vi "test2-TestFilterJKISMStringQueueVI.vi"(8 "error in (no error)":errorcluster, 11 "TestCase in":refnum<class "testcase-CSMManagementAPI.lvclass">) -> (0 "error out":errorcluster, 3 "TestCase out":refnum<class "testcase-CSMManagementAPI.lvclass">)   [LabVIEW 2017, in "testcase-CSMManagementAPI.lvclass"]
uses:
  testcase-CSMManagementAPI.lvclass
  src/user.lib/_NEVSTOP/Communicable State Machine(CSM)/AdvanceAPI/CSM - Revert Arguments-Safe String.vi
  src/user.lib/_NEVSTOP/Communicable State Machine(CSM)/AdvanceAPI/CSM - Make String Arguments Safe.vi
  src/user.lib/_NEVSTOP/Communicable State Machine(CSM)/AdvanceAPI/CSM - Break Down Multiple States String.vi
  src/user.lib/_NEVSTOP/Communicable State Machine(CSM)/AdvanceAPI/CSM - Compact Multiple States.vi
  src/user.lib/_NEVSTOP/Communicable State Machine(CSM)/AdvanceAPI/CSM - Keywords.vi
  src/user.lib/_NEVSTOP/Communicable State Machine(CSM)/_Polymophic/CSM - Filter Interrupt Broadcasts.vi
  src/user.lib/_NEVSTOP/Communicable State Machine(CSM)/_Polymophic/CSM - Filter Status Broadcasts.vi
  src/user.lib/_NEVSTOP/Communicable State Machine(CSM)/_Polymophic/CSM - Filter Broadcasts.vi
  src/user.lib/_NEVSTOP/Communicable State Machine(CSM)/_Polymophic/CSM - Filter Sync Messages.vi
  src/user.lib/_NEVSTOP/Communicable State Machine(CSM)/_Polymophic/CSM - Filter Async without Reply Messages.vi
  src/user.lib/_NEVSTOP/Communicable State Machine(CSM)/_Polymophic/CSM - Filter Async Messages.vi
  src/user.lib/_NEVSTOP/Communicable State Machine(CSM)/_Polymophic/CSM - Filter Messges.vi
  src/user.lib/_NEVSTOP/Communicable State Machine(CSM)/_Polymophic/CSM - Filter Local States.vi
  src/user.lib/_NEVSTOP/Communicable State Machine(CSM)/_Polymophic/CSM - Filter Duplicated Lines.vi
  src/user.lib/_NEVSTOP/Communicable State Machine(CSM)/AdvanceAPI/CSM - Filter Messages to Non-Existing Modules.vi
  src/user.lib/_NEVSTOP/Communicable State Machine(CSM)/_Shared/Trim Single-line Text.vi
  <vilib>/addons/_JKI Toolkits/VI Tester/TestCase.llb/TestCase.lvclass
  src/user.lib/_NEVSTOP/Communicable State Machine(CSM)/Communicable State Machine.lvlib
  C:/Program Files (x86)/National Instruments/LabVIEW 2017/vi.lib/addons/_JKI Toolkits/VI Tester/TestCase.llb/TestCase.lvclass
panel:
  out "Filter Duplicate Lines No Comments":bool
  out "Filter Duplicate Lines":bool
  out "Filter Duplicate States(Regardless of async/sync/status/interrupt)":bool
  out "Fiter Interrupt Broadcast":bool
  out "Fiter Status Broadcast":bool
  out "Fiter Broadcasts":bool
  out "Filter Messages To Non Existing CSMs":bool
  out "Filter Sync Messages":bool
  out "Filter Async Messages Without Reply":bool
  out "Filter Async Messages":bool
  out "Filter All Messages":bool
  out "Fiter Local States":bool
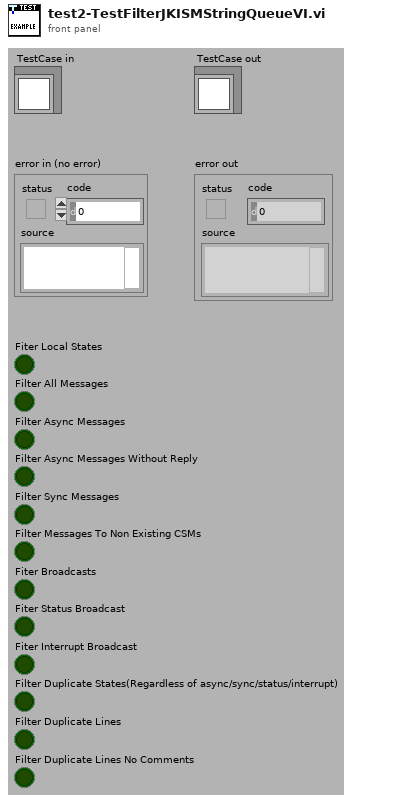
[diagram p1: front panel]
types:
  T1 = enum32{"Invalid", "Standard", "Closed", "Hidden", "Minimized", "Maximized"}
  T2 = enum32{"invalid app kind", "Development System", "Run Time System", "Student Edition", "Embedded LabVIEW", "Evaluation", "Custom"}
  T3 = typedef "Communicable State Machine.lvlib/_CSM_Response Source Message.ctl" = cluster{"‘State":string, "’Arguments":string, "’Error":errorcluster}
  T4 = cluster{"Current VI Reference":refnum<vi>, "Close Panel on Exit?":bool}
  T5 = cluster{"Core":cluster{"Current VI Reference":refnum<vi>, "Close Panel on Exit?":bool}, "Your Boolean data":bool, "Your string data":string}
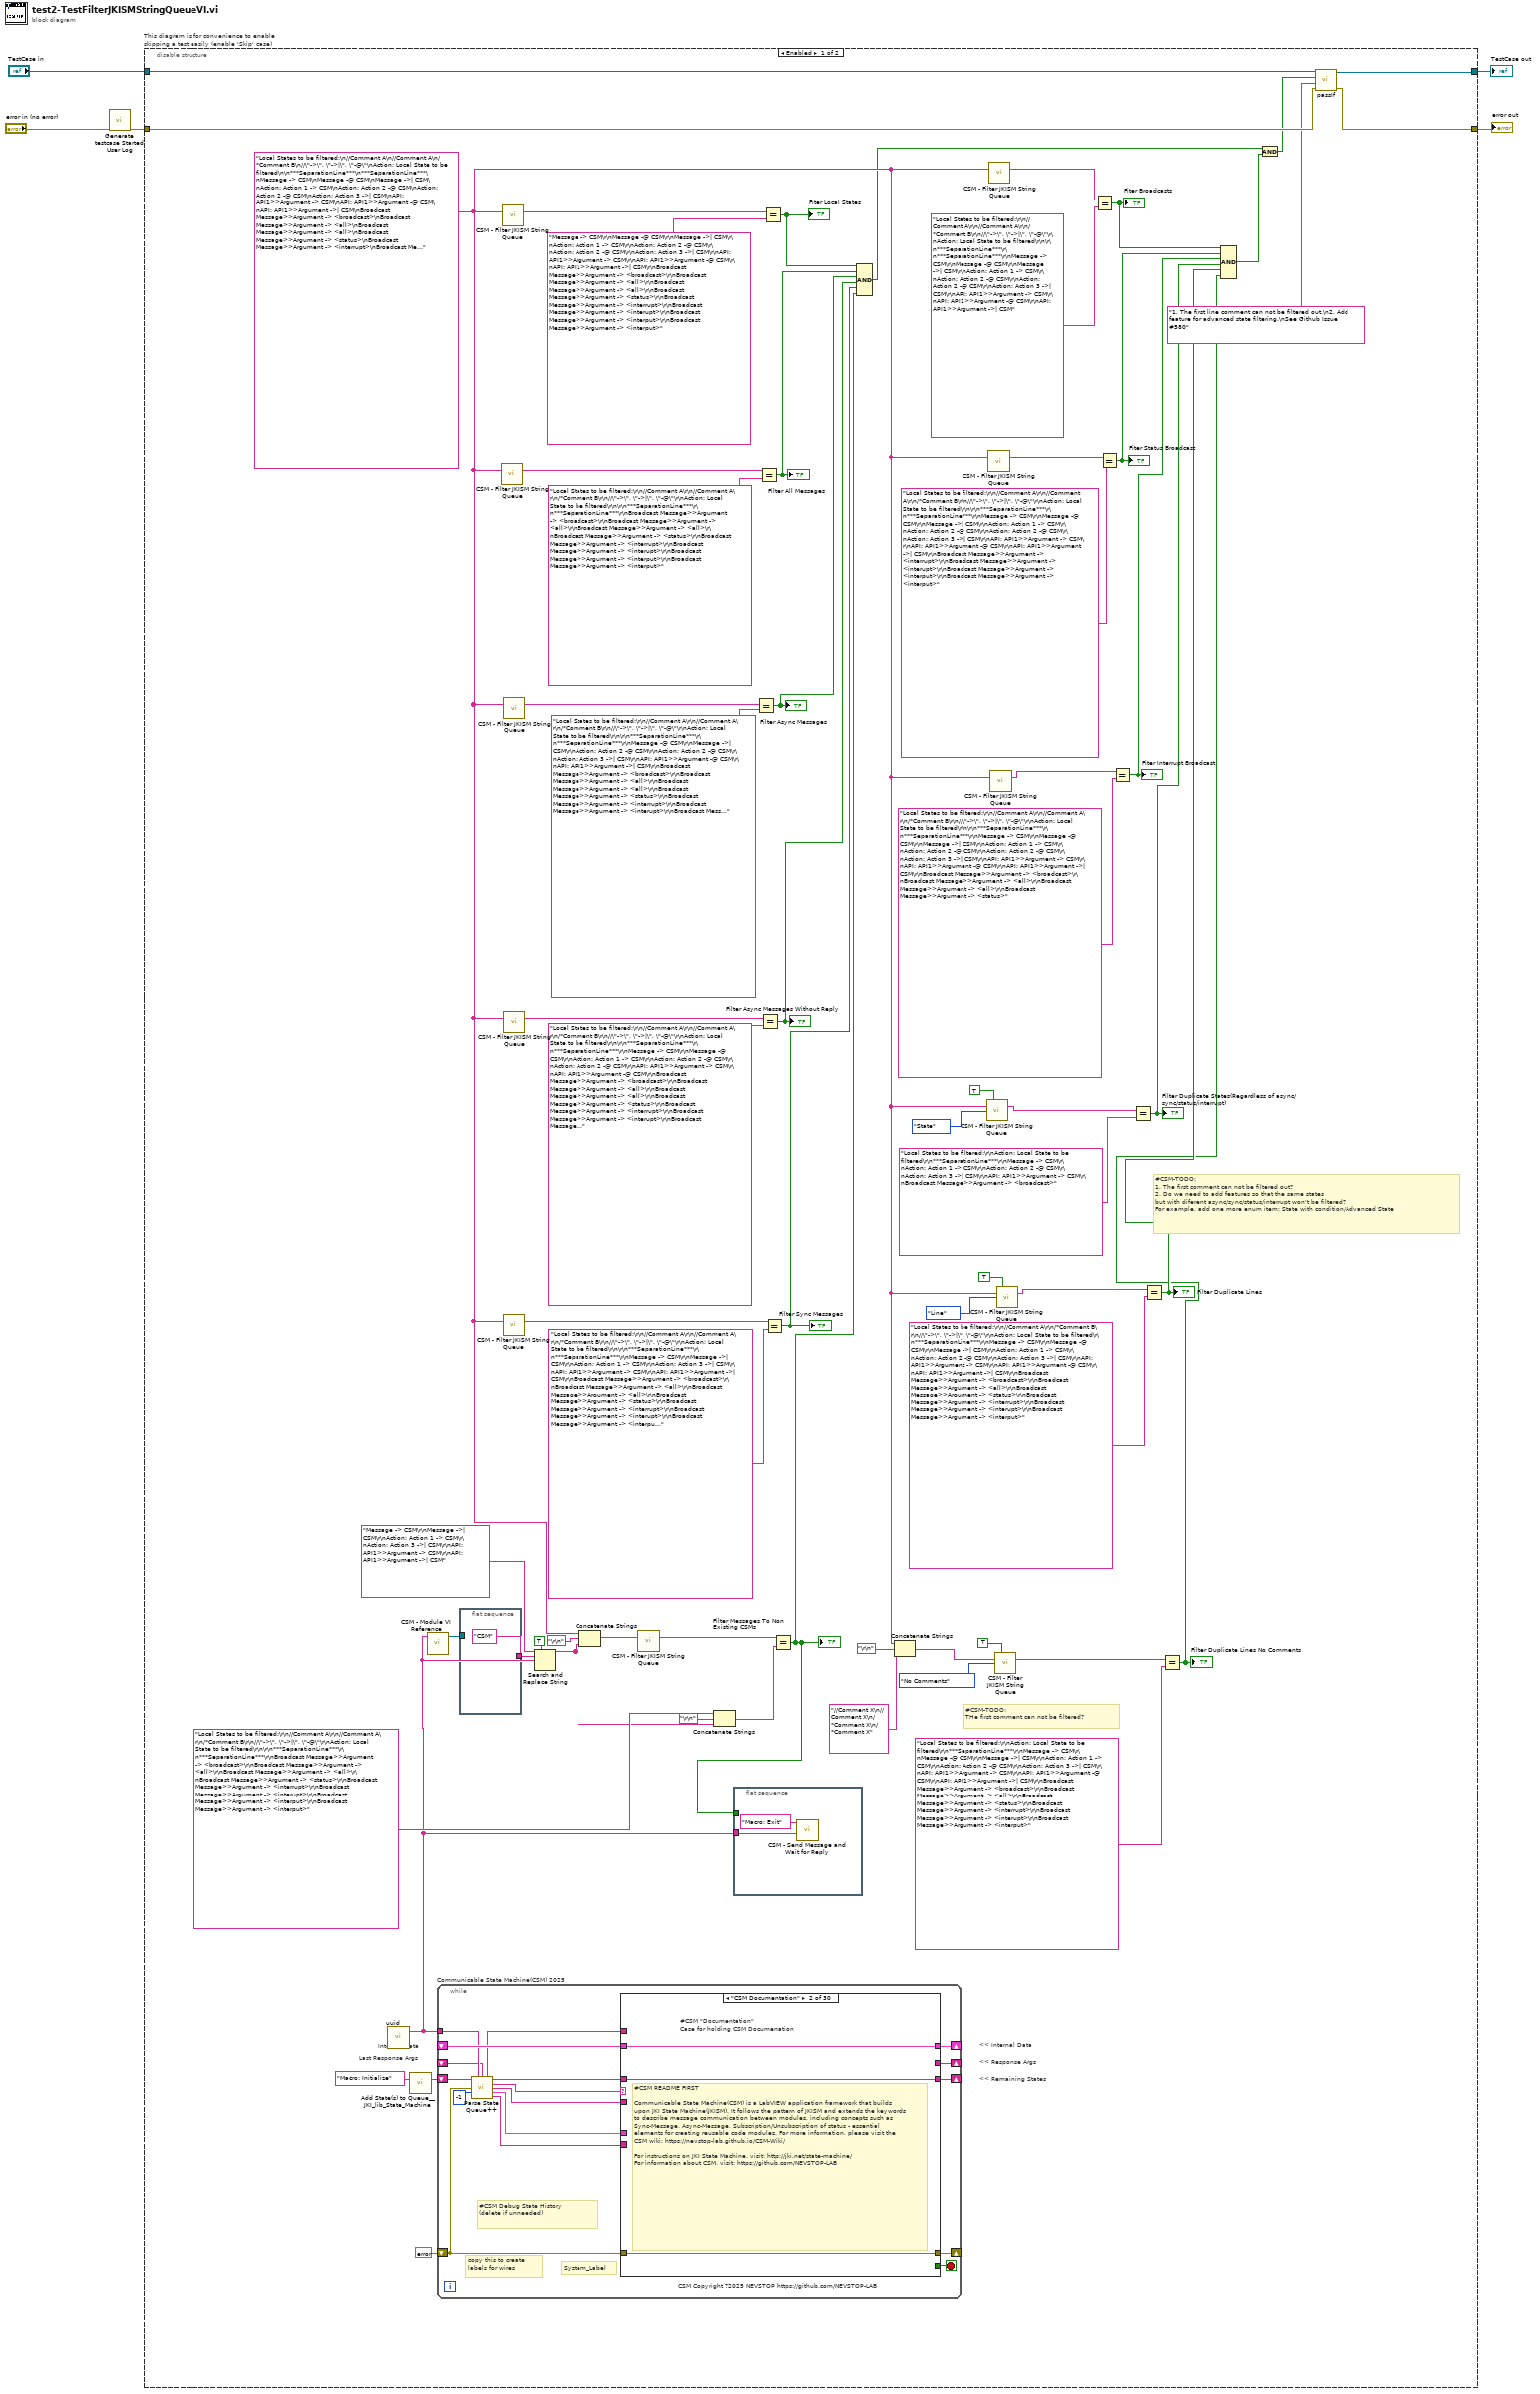
[diagram p0: block diagram]
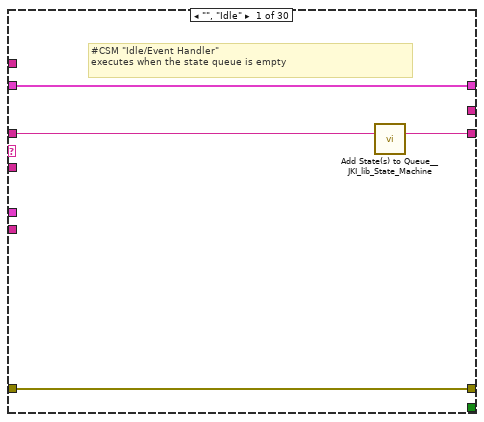
[diagram p2: hidden frame]
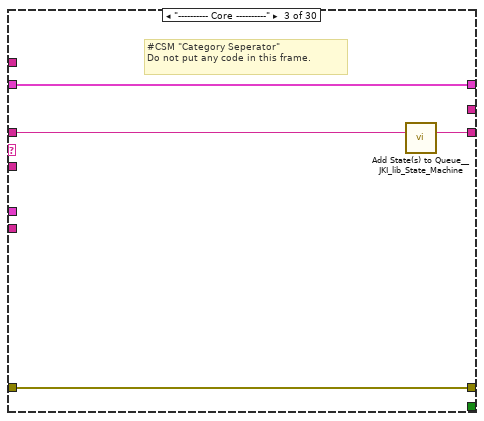
[diagram p3: hidden frame]
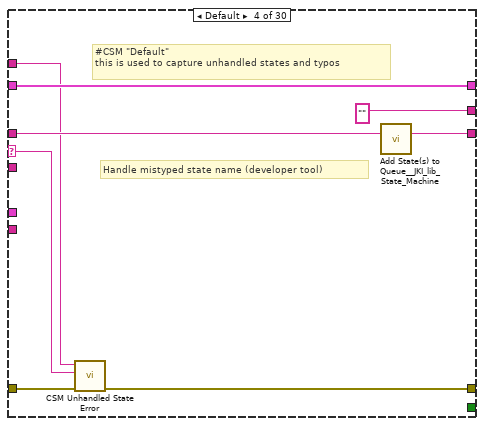
[diagram p4: hidden frame]
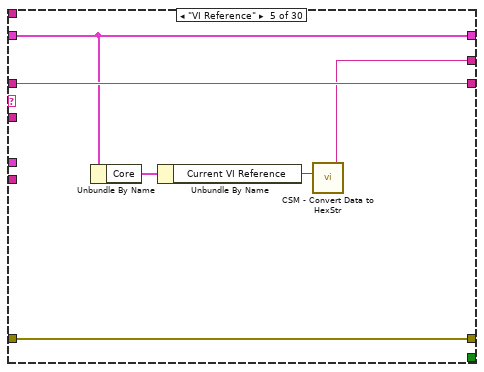
[diagram p5: hidden frame]
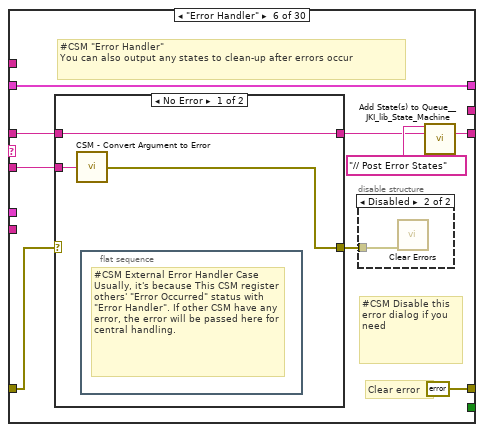
[diagram p6: hidden frame]
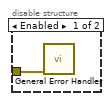
[diagram p7: hidden frame]
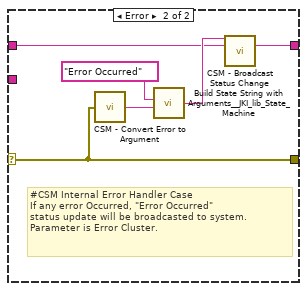
[diagram p8: hidden frame]
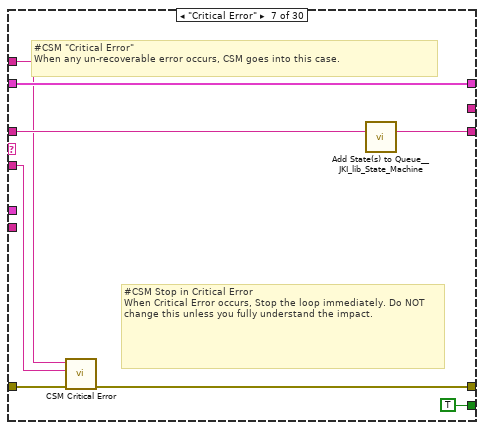
[diagram p9: hidden frame]
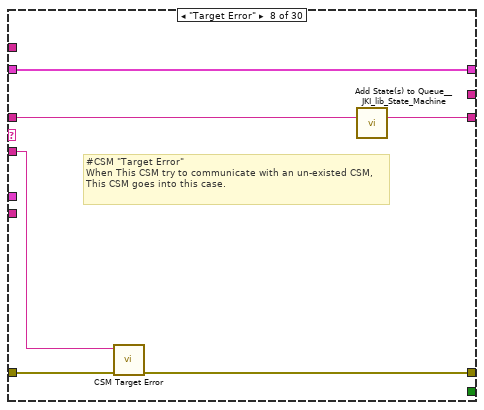
[diagram p10: hidden frame]
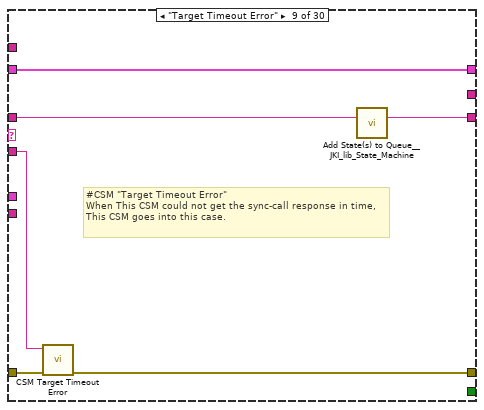
[diagram p11: hidden frame]
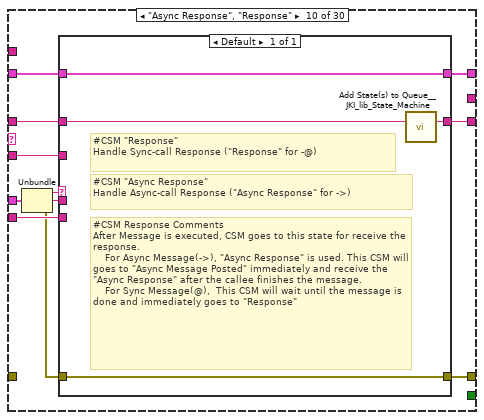
[diagram p12: hidden frame]
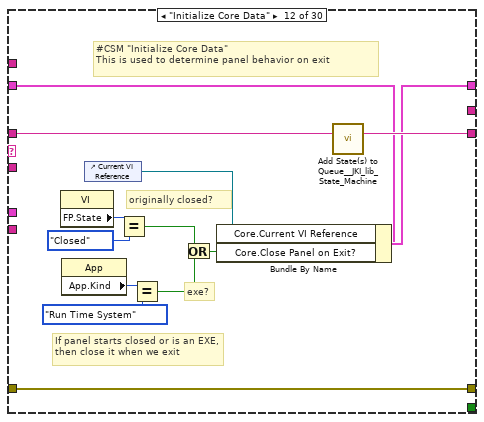
[diagram p14: hidden frame]
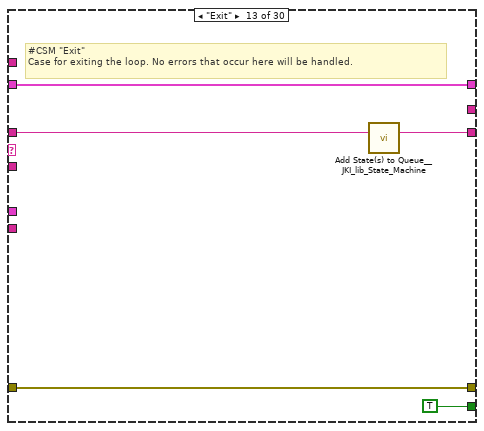
[diagram p15: hidden frame]
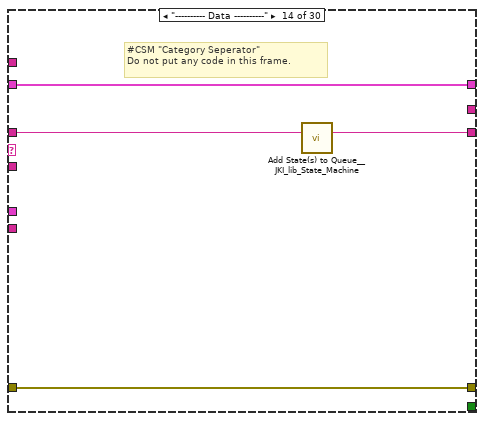
[diagram p16: hidden frame]
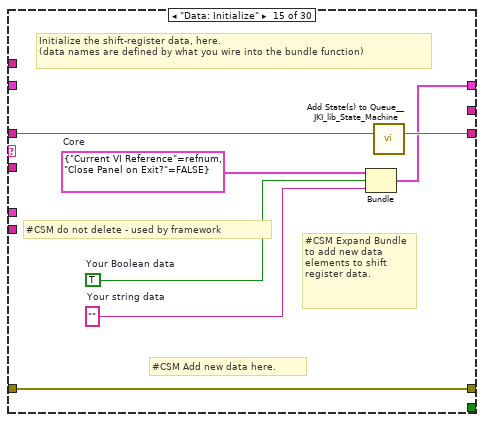
[diagram p17: hidden frame]
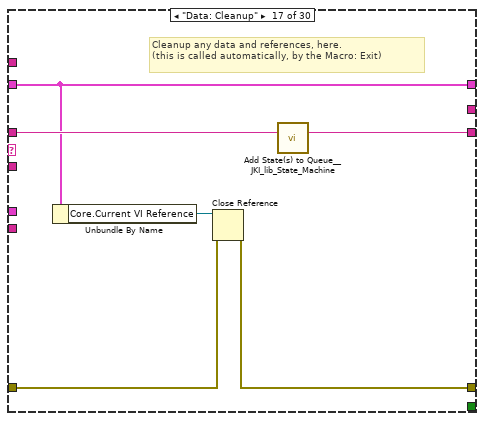
[diagram p19: hidden frame]
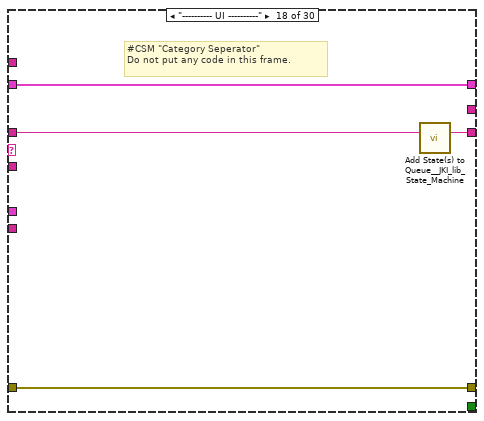
[diagram p20: hidden frame]
diagram:
  n1 = call "Generate testcase Started User Log.vi"("Error In"="error in (no error)") -> ("error out"=w1:errorcluster)  [unwired: 10 in]
  n2 = disable-structure "This diagram is for convenience to enable skipping a test easily (enable 'Skip' case)" shown="Enabled" {
    disable-tunnel: "TestCase in" -> [w32 w353]
    disable-tunnel: [w33 w351] -> w2
    disable-tunnel: [w30 w352] -> w4
    disable-tunnel: w1 -> [w31 w350]
    frame Enabled {
      w38 = "Local States to be filtered:\n//Comment A\n//Comment A\n/*Comment B\n//\"->\", \"->|\", \"-@\"\nAction: Local State to be filtered\n\n***SeparationLine***\n***SeparationLine***\nMessage -> CSM\nMessage -@ CSM\nMessage ->| CSM\nAction: Action 1 -> CSM\nAction: Action 2 -@ CSM\nAction: Action 2 -@ CSM\nAction: Action 3 ->| CSM\nAPI: API1>>Argument -> CSM\nAPI: API1>>Argument -@ CSM\nAPI: API1>>Argument ->| CSM\nBroadcast Message>>Argument -> <broadcast>\nBroadcast Message>>Argument -> <all>\nBroadcast Message>>Argument -> <all>\nBroadcast Message>>Argument -> <status>\nBroadcast Message>>Argument -> <interrupt>\nBroadcast Message>>Argument -> <interupt>\nBroadcast Message>>Argument -> <interput>\nBroadcast Message>>Argument -> <interput>" ("States In")
      # "Last Response Args"
      # "Internal Data"
      # "<< Internal Data"
      # "<< Response Args"
      # "<< Remaining States"
      # "#CSM-TODO:\nTHe first comment can not be filtered?"
      # "#CSM-TODO:\n1. The first comment can not be filtered out?\n2. Do we need to add features so that the same states \nbut with diferent async/sync/status/interrupt won't be filtered?\nFor example, add one more enum item: State with condition/Advanced State"
      n3 = call "uuid.vi"() -> ("UUID"=w7:string)  [unwired: 11 in]
      n4 = call <vilib>:"Add State(s) to Queue__JKI_lib_State_Machine.vi"("State(s) in (\"\")"="Macro: Initialize" ("Init State(\"Macro: Initialize\")")) -> ("States Out"=w11:string)  [unwired: 14 in]
      n5 = call "CSM - Module VI Reference.vi"("CSM Name"=w7) -> ("CSM Module VIRef"=w8:refnum<vi>)  [unwired: 9 in, 1 out]
      n6 = while "Communicable State Machine(CSM) 2025" {
        shift-right: [w87] -> _
        shift-left: _ -> [w86]
        shift-right: [w90] -> _
        shift-left: errorcluster {"status"=FALSE, "code"=0, "source"=""} ("error out") -> [w85]
        shift-right: [w89] -> _
        shift-left: w11 -> [w91]
        tunnel: w7 -> [w83]
        shift-right: [w84] -> _
        shift-left: _ -> [w77]
        stop <- w88 stop-if-true
        # "#CSM Debug State History\n(delete if unneeded)"
        # "copy this to create labels for wires"
        # "System_Label"
        # "CSM Copyright ?2025 NEVSTOP https://github.com/NEVSTOP-LAB"
        n7 = call "Parse State Queue++.vi"("State Queue"=w91, "Name (\"\" to Use UUID)"=w83, "Response Arguments"=w77, "Previous Error"=w85, "Dequeue (1 ms)"=-1 ("Timeout")) -> ("Name Used"=w78:string, "Remaining States"=w92:string, "Current State"=w82:string, "Arguments"=w81:string, "Additional Information"=w80:T3, "Source CSM"=w79:string)  [unwired: 5 in]
        n8 = case shown="\"CSM Documentation\"" w82 {
          selector: w82 -> [_ _ _ w106 _ _ _ _ _ _ _ _ _ _ _ _ _ _ _ _ _ _ _ _ _ _ _ _ _ _]
          tunnel: w92 -> [w93 w98 w103 w110 w116 w122 w143 w149 w155 w163 w174 w188 w193 w197 w204 w206 w213 w217 w221 w227 w242 w311 w316 w323 w325 w329 w334 w341 w345 w349]
          tunnel: w81 -> [_ _ _ _ _ w121 w139 w148 w153 w162 _ _ _ _ _ _ _ _ _ w222 w236 _ _ _ _ _ w332 _ _ _]
          tunnel: w86 -> [w94 w97 w100 w108 w115 w125 w144 w150 w156 w165 w173 w181 w191 w194 _ w205 w208 w214 w219 w225 w238 w308 w313 w320 w324 w328 w333 w338 w342 w346]
          tunnel: [w95 w99 w101 w104 w117 errorcluster {"status"=FALSE, "code"=0, "source"=""} ("error out") w140 w146 w152 w168 w175 w185 w190 w195 w201 w207 w209 w215 w218 w223 w239 w309 w314 w321 w326 w330 w335 w339 w343 w347] -> w90
          tunnel: w85 -> [w95 w99 w101 w111 w117 w123 w145 w147 w154 _ w175 w185 w190 w195 w201 w207 w210 w215 w218 w224 w240 w309 w314 w321 w326 w330 w335 w339 w343 w347]
          tunnel: [w96 w98 w102 w109 w116 w118 w142 w151 w157 w164 w174 w187 w192 w196 w203 w206 w212 w216 w220 w226 w241 w310 w315 w322 w325 w329 w334 w340 w344 w348] -> w89
          tunnel: [_ _ _ _ _ _ TRUE _ _ _ _ _ TRUE _ _ _ _ _ _ _ _ _ _ _ _ _ _ _ _ _] -> w88
          tunnel: [w94 w97 w100 w108 w115 w125 w144 w150 w156 w166 w173 w186 w191 w194 w202 w205 w208 w214 w219 w225 w238 w308 w313 w320 w324 w328 w333 w338 w342 w346] -> w87
          tunnel: w79 -> [_ _ _ _ _ _ _ _ _ w160 _ _ _ _ _ _ _ _ _ _ _ _ _ _ _ _ _ _ _ _]
          tunnel: w80 -> [_ _ _ _ _ _ _ _ _ w167 _ _ _ _ _ _ _ _ _ _ _ _ _ _ _ _ _ _ _ _]
          tunnel: [_ _ _ "" w112 _ _ _ _ _ _ _ _ _ _ _ _ _ _ _ _ _ _ _ _ "API1 Response" w331 _ _ _] -> w84
          tunnel: w78 -> [_ _ _ w105 _ _ w138 _ _ _ _ _ _ _ _ _ _ _ _ _ _ _ _ _ _ _ _ _ _ _]
          frame "", "Idle" {
            # "#CSM \"Idle/Event Handler\"\nexecutes when the state queue is empty"
            n9 = call <vilib>:"Add State(s) to Queue__JKI_lib_State_Machine.vi"("State(s) in (\"\")"=w93) -> ("States Out"=w96:string)  [unwired: 14 in]
          }
          frame "CSM Documentation" {
            # "#CSM README FIRST\n\nCommunicable State Machine(CSM) is a LabVIEW application framework that builds upon JKI State Machine(JKISM). It follows the pattern of JKISM and extends the keywords to describe message communication between modules, including concepts such as Sync-Message, Async-Message, Subscription/Unsubscription of status - essential elements for creating reusable code modules. For more information, please visit the CSM wiki: https://nevstop-lab.github.io/CSM-Wiki/\n\nFor instructions on JKI State Machine, visit: http://jki.net/state-machine/\nFor information about CSM, visit: https://github.com/NEVSTOP-LAB"
            # "#CSM \"Documentation\"\nCase for holding CSM Documenation"
          }
          frame "---------- Core ----------" {
            # "#CSM \"Category Seperator\"\nDo not put any code in this frame."
            n10 = call <vilib>:"Add State(s) to Queue__JKI_lib_State_Machine.vi"("State(s) in (\"\")"=w103) -> ("States Out"=w102:string)  [unwired: 14 in]
          }
          frame Default {
            # "#CSM \"Default\"\nthis is used to capture unhandled states and typos"
            # "Handle mistyped state name (developer tool)"
            n11 = call "CSM Unhandled State Error.vi"("error in (no error)"=w111, "Undefined State"=w106, "CSM Name"=w105) -> ("error out"=w104:errorcluster)  [unwired: 8 in]
            n12 = call <vilib>:"Add State(s) to Queue__JKI_lib_State_Machine.vi"("State(s) in (\"\")"=w110) -> ("States Out"=w109:string)  [unwired: 14 in]
          }
          frame "VI Reference" {
            n13 = Unbundle By Name(w115) -> ("Core"=w114:T4)
            n14 = Unbundle By Name(w114) -> ("Current VI Reference"=w113:refnum<vi>)
            n15 = call "CSM - Convert Data to HexStr.vi"("Variant"=w113) -> ("HEX String (0-9,A-F)"=w112:string)  [unwired: 8 in]
          }
          frame "Error Handler" {
            # "#CSM Disable this error dialog if you need"
            # "#CSM \"Error Handler\"\nYou can also output any states to clean-up after errors occur"
            # "Clear error"
            n16 = case shown="No Error" w123 {
              selector: w123 -> [_ w132]
              tunnel: [w131 w134] -> w119
              tunnel: w122 -> [w131 w133]
              tunnel: w121 -> [w130 _]
              tunnel: [w129 w132] -> w124
              frame No Error {
                n17 = call "CSM - Convert Argument to Error.vi"("Argument"=w130) -> ("Error"=w129:errorcluster)  [unwired: 4 in]
                n18 = flat-sequence {
                  frame #0 {
                    # "#CSM External Error Handler Case\nUsually, it's because This CSM register others' \"Error Occurred\" status with \"Error Handler\". If other CSM have any error, the error will be passed here for central handling."
                  }
                }
              }
              frame Error {
                # "#CSM Internal Error Handler Case \nIf any error Occurred, \"Error Occurred\" \nstatus update will be broadcasted to system.\nParameter is Error Cluster."
                n19 = call "CSM - Convert Error to Argument.vi"("Error"=w132) -> ("Argument"=w136:string)  [unwired: 4 in]
                n20 = call <vilib>:"Build State String with Arguments__JKI_lib_State_Machine.vi"("Arguments (\"\")"=w136, "State"="Error Occurred" ("Status with Arguments")) -> ("State with Arguments"=w135:string)  [unwired: 4 in]
                n21 = call "CSM - Broadcast Status Change.vi"("Status With Arguments"=w135, "State Queue"=w133) -> ("Remaining States"=w134:string)  [unwired: 13 in]
              }
            }
            n22 = disable-structure shown="Disabled" {
              disable-tunnel: w124 -> [w127 w128]
              frame Enabled {
                n23 = call <vilib>:"General Error Handler.vi"("error in (no error)"=w127) -> ()  [unwired: 10 in, 5 out]
              }
              frame Disabled {
                n24 = call <vilib>:"Clear Errors.vi"("error in (no error)"=w128) -> ()  [unwired: 5 in, 2 out]
              }
            }
            n25 = call <vilib>:"Add State(s) to Queue__JKI_lib_State_Machine.vi"("State(s) in Front (\"\")"="// Post Error States", "State(s) in (\"\")"=w119) -> ("States Out"=w118:string)  [unwired: 13 in]
          }
          frame "Critical Error" {
            # "#CSM Stop in Critical Error\nWhen Critical Error occurs, Stop the loop immediately. Do NOT change this unless you fully understand the impact."
            # "#CSM \"Critical Error\"\nWhen any un-recoverable error occurs, CSM goes into this case."
            n26 = call "CSM Critical Error.vi"("error in (no error)"=w145, "Arugments (As Reason)"=w139, "CSM Name"=w138) -> ("error out"=w140:errorcluster)  [unwired: 8 in]
            n27 = call <vilib>:"Add State(s) to Queue__JKI_lib_State_Machine.vi"("State(s) in (\"\")"=w143) -> ("States Out"=w142:string)  [unwired: 14 in]
          }
          frame "Target Error" {
            # "#CSM \"Target Error\"\nWhen This CSM try to communicate with an un-existed CSM, This CSM goes into this case."
            n28 = call "CSM Target Error.vi"("error in (no error)"=w147, "Arguments (As CSM Name)"=w148) -> ("error out"=w146:errorcluster)  [unwired: 9 in]
            n29 = call <vilib>:"Add State(s) to Queue__JKI_lib_State_Machine.vi"("State(s) in (\"\")"=w149) -> ("States Out"=w151:string)  [unwired: 14 in]
          }
          frame "Target Timeout Error" {
            # "#CSM \"Target Timeout Error\"\nWhen This CSM could not get the sync-call response in time, This CSM goes into this case."
            n30 = call "CSM Target Timeout Error.vi"("error in (no error)"=w154, "Arguments (As CSM Name)"=w153) -> ("error out"=w152:errorcluster)  [unwired: 9 in]
            n31 = call <vilib>:"Add State(s) to Queue__JKI_lib_State_Machine.vi"("State(s) in (\"\")"=w155) -> ("States Out"=w157:string)  [unwired: 14 in]
          }
          frame "Async Response", "Response" {
            n32 = Unbundle(w167) -> ("‘State"=w161:string, "’Arguments"=w159:string, "’Error"=w158:errorcluster)
            n33 = case shown="Default" w161 {
              tunnel: [w172] -> w168
              tunnel: w158 -> [w172]
              tunnel: [w171] -> w166
              tunnel: w165 -> [w171]
              tunnel: [w169] -> w164
              tunnel: w163 -> [w170]
              tunnel: w162 -> [_]
              tunnel: w160 -> [_]
              tunnel: w159 -> [_]
              frame Default {
                # "#CSM Response Comments\nAfter Message is executed, CSM goes to this state for receive the response.\n    For Async Message(->), \"Async Response\" is used. This CSM will goes to \"Async Message Posted\" immediately and receive the \"Async Response\" after the callee finishes the message.\n    For Sync Message(@),  This CSM will wait until the message is done and immediately goes to \"Response\""
                # "#CSM \"Async Response\"\nHandle Async-call Response (\"Async Response\" for ->)"
                # "#CSM \"Response\"\nHandle Sync-call Response (\"Response\" for -@)"
                n34 = call <vilib>:"Add State(s) to Queue__JKI_lib_State_Machine.vi"("State(s) in (\"\")"=w170) -> ("States Out"=w169:string)  [unwired: 14 in]
              }
            }
          }
          frame "Async Message Posted" {
            # "#CSM \"Async Message Posted\"\nAfter Async Message is posted (-> or ->| ), CSM goes to this state for post-action.\nYou can use Argument - State to tell which Async Message is called."
          }
          frame "Initialize Core Data" {
            # "#CSM \"Initialize Core Data\"\nThis is used to determine panel behavior on exit"
            # "originally closed?"
            # "exe?"
            # "If panel starts closed or is an EXE, then close it when we exit"
            n35 = property class="VI"() -> ("FP.State"=w178:T1)  [unwired: 2 in, 2 out]
            n36 = property class="App"() -> ("App.Kind"=w184:T2)  [unwired: 2 in, 2 out]
            n37 = control-ref of="Current VI Reference"() -> (w179:refnum<vi>)
            n38 = Equal?(x=w178, y=T1."Closed" ("Front Panel Window:State")) -> (x = y?=w176:bool)
            n39 = Equal?(x=w184, y=T2."Run Time System" ("Application:Kind")) -> (x = y?=w182:bool)
            n40 = Or(x=w176, y=w182) -> (x .or. y?=w180:bool)
            n41 = Bundle By Name(cluster=w181, "Core.Current VI Reference"=w179, "Core.Close Panel on Exit?"=w180) -> (w186:T5)
            n42 = call <vilib>:"Add State(s) to Queue__JKI_lib_State_Machine.vi"("State(s) in (\"\")"=w188) -> ("States Out"=w187:string)  [unwired: 14 in]
          }
          frame "Exit" {
            # "#CSM \"Exit\"\nCase for exiting the loop. No errors that occur here will be handled."
            n43 = call <vilib>:"Add State(s) to Queue__JKI_lib_State_Machine.vi"("State(s) in (\"\")"=w193) -> ("States Out"=w192:string)  [unwired: 14 in]
          }
          frame "---------- Data ----------" {
            # "#CSM \"Category Seperator\"\nDo not put any code in this frame."
            n44 = call <vilib>:"Add State(s) to Queue__JKI_lib_State_Machine.vi"("State(s) in (\"\")"=w197) -> ("States Out"=w196:string)  [unwired: 14 in]
          }
          frame "Data: Initialize" {
            w198 = T4 {"Current VI Reference"=refnum, "Close Panel on Exit?"=FALSE}  # Core
            w200 = TRUE  # Your Boolean data
            w199 = ""  # Your string data
            # "#CSM do not delete - used by framework"
            # "#CSM Expand Bundle to add new data elements to shift register data."
            # "#CSM Add new data here."
            # "Initialize the shift-register data, here.\n(data names are defined by what you wire into the bundle function)"
            n45 = Bundle("Core"=w198, "Your Boolean data"=w200, "Your string data"=w199) -> (w202:T5)  [unwired: 1 in]
            n46 = call <vilib>:"Add State(s) to Queue__JKI_lib_State_Machine.vi"("State(s) in (\"\")"=w204) -> ("States Out"=w203:string)  [unwired: 14 in]
          }
          frame "Data: Update Indicators" {
          }
          frame "Data: Cleanup" {
            # "Cleanup any data and references, here.\n(this is called automatically, by the Macro: Exit)"
            n47 = Unbundle By Name(w208) -> ("Core.Current VI Reference"=w211:refnum<vi>)
            n48 = Close Reference(reference=w211, error in (no error)=w210) -> (error out=w209:errorcluster)
            n49 = call <vilib>:"Add State(s) to Queue__JKI_lib_State_Machine.vi"("State(s) in (\"\")"=w213) -> ("States Out"=w212:string)  [unwired: 14 in]
          }
          frame "---------- UI ----------" {
            # "#CSM \"Category Seperator\"\nDo not put any code in this frame."
            n50 = call <vilib>:"Add State(s) to Queue__JKI_lib_State_Machine.vi"("State(s) in (\"\")"=w217) -> ("States Out"=w216:string)  [unwired: 14 in]
          }
          frame "UI: Initialize" {
            # "#CSM \"UI: Initialize\"\nInitialize the User Interface, here.\n(this is called automatically, by the Macro: Init)"
            n51 = call <vilib>:"Add State(s) to Queue__JKI_lib_State_Machine.vi"("State(s) in (\"\")"=w221) -> ("States Out"=w220:string)  [unwired: 14 in]
          }
          frame "UI: Cursor Set" {
            # "#CSM \"UI: Cursor Set\"\nSet and Unset Cursor Busy.\n(Usage: \"UI: Cursor Set >> Busy|Idle\")"
            # "Argument"
            n52 = disable-structure shown="TARGET_TYPE!=Windows" {
              disable-tunnel: w224 -> [w230 w235]
              disable-tunnel: [w229 w235] -> w223
              disable-tunnel: w222 -> [w228 _]
              frame condition #0 (active) {
                n53 = case shown="\"Idle\", Default" w228 {
                  tunnel: w230 -> [w232 w234]
                  tunnel: [w231 w233] -> w229
                  frame "Idle", Default {
                    n54 = call <vilib>:"Unset Busy.vi"("error in (no error)"=w232) -> ("error out"=w231:errorcluster)  [unwired: 10 in]
                  }
                  frame "Busy" {
                    n55 = call <vilib>:"Set Busy.vi"("error in (no error)"=w234) -> ("error out"=w233:errorcluster)  [unwired: 9 in, 1 out]
                  }
                }
              }
              frame condition #1 {
              }
            }
            n56 = call <vilib>:"Add State(s) to Queue__JKI_lib_State_Machine.vi"("State(s) in (\"\")"=w227) -> ("States Out"=w226:string)  [unwired: 14 in]
          }
          frame "UI: Front Panel State" {
            # "#CSM \"UI: Front Panel State\"\nSet Front Panel Open or Closed\n(Usage: \"UI: Front Panel State >> Open|Close\")"
            # "Argument"
            n57 = Unbundle By Name(w238) -> ("Core.Current VI Reference"=w237:refnum<vi>)
            n58 = call <vilib>:"Add State(s) to Queue__JKI_lib_State_Machine.vi"("State(s) in (\"\")"=w242) -> ("States Out"=w241:string)  [unwired: 14 in]
            n59 = case shown="\"Close\", \"Closed\"" w236 {
              tunnel: w240 -> [w248 w263 w274 w287 w300]
              tunnel: [w250 w264 w276 w289 w302] -> w239
              tunnel: w237 -> [w249 w261 w275 w288 w301]
              frame "Open", "Standard", Default {
                w243 = T1."Standard" ("State")
                n60 = property class="VI"(reference=w249, error in=w248) -> (reference out=w246:refnum<vi>, error out=w247:errorcluster, "FP.State"=w245:T1)
                n61 = Not Equal?(x=w245, y=w243) -> (x != y?=w244:bool)
                n62 = case shown="True" w244 {
                  tunnel: [w254 w256] -> w250
                  tunnel: w247 -> [w253 w256]
                  tunnel: w246 -> [w252 _]
                  tunnel: w243 -> [w251 _]
                  frame True {
                    n63 = invoke class="VI" method="FP.Open"(reference=w252, error in=w253, "Activate"=TRUE, "State"=w251) -> (error out=w254:errorcluster)  [unwired: 1 in, 4 out]
                  }
                  frame False {
                  }
                }
              }
              frame "Close", "Closed" {
                n64 = property class="VI"(reference=w261, error in=w263) -> (reference out=w260:refnum<vi>, error out=w262:errorcluster, "FP.State"=w258:T1)
                n65 = Not Equal?(x=w258, y=T1."Closed" ("Front Panel Window:State")) -> (x != y?=w257:bool)
                n66 = case shown="False" w257 {
                  tunnel: [w265 w268] -> w264
                  tunnel: w262 -> [w265 w267]
                  tunnel: w260 -> [_ w266]
                  frame False {
                  }
                  frame True {
                    n67 = invoke class="VI" method="FP.Close"(reference=w266, error in=w267) -> (error out=w268:errorcluster)  [unwired: 1 in, 2 out]
                  }
                }
              }
              frame "Hidden", "Hide" {
                w269 = T1."Hidden" ("State")
                n68 = property class="VI"(reference=w275, error in=w274) -> (reference out=w272:refnum<vi>, error out=w273:errorcluster, "FP.State"=w271:T1)
                n69 = Not Equal?(x=w271, y=w269) -> (x != y?=w270:bool)
                n70 = case shown="True" w270 {
                  tunnel: [w280 w281] -> w276
                  tunnel: w273 -> [w279 w281]
                  tunnel: w272 -> [w278 _]
                  tunnel: w269 -> [w277 _]
                  frame True {
                    n71 = invoke class="VI" method="FP.Open"(reference=w278, error in=w279, "State"=w277) -> (error out=w280:errorcluster)  [unwired: 2 in, 4 out]
                  }
                  frame False {
                  }
                }
              }
              frame "Minimize", "Minimized" {
                w282 = T1."Minimized" ("State")
                n72 = property class="VI"(reference=w288, error in=w287) -> (reference out=w285:refnum<vi>, error out=w286:errorcluster, "FP.State"=w284:T1)
                n73 = Not Equal?(x=w284, y=w282) -> (x != y?=w283:bool)
                n74 = case shown="True" w283 {
                  tunnel: [w293 w294] -> w289
                  tunnel: w286 -> [w292 w294]
                  tunnel: w285 -> [w291 _]
                  tunnel: w282 -> [w290 _]
                  frame True {
                    n75 = invoke class="VI" method="FP.Open"(reference=w291, error in=w292, "State"=w290) -> (error out=w293:errorcluster)  [unwired: 2 in, 4 out]
                  }
                  frame False {
                  }
                }
              }
              frame "Maximize", "Maximized" {
                w295 = T1."Maximized" ("State")
                n76 = property class="VI"(reference=w301, error in=w300) -> (reference out=w298:refnum<vi>, error out=w299:errorcluster, "FP.State"=w297:T1)
                n77 = Not Equal?(x=w297, y=w295) -> (x != y?=w296:bool)
                n78 = case shown="True" w296 {
                  tunnel: [w306 w307] -> w302
                  tunnel: w299 -> [w305 w307]
                  tunnel: w298 -> [w304 _]
                  tunnel: w295 -> [w303 _]
                  frame True {
                    n79 = invoke class="VI" method="FP.Open"(reference=w304, error in=w305, "State"=w303) -> (error out=w306:errorcluster)  [unwired: 2 in, 4 out]
                  }
                  frame False {
                  }
                }
              }
            }
          }
          frame "---------- Macro ----------" {
            # "#CSM \"Category Seperator\"\nDo not put any code in this frame."
            n80 = call <vilib>:"Add State(s) to Queue__JKI_lib_State_Machine.vi"("State(s) in (\"\")"=w311) -> ("States Out"=w310:string)  [unwired: 14 in]
          }
          frame "Macro: Initialize" {
            # "#CSM \"Macro: Initialize\"\nInitialization Macro (This is called once, when the VI starts)"
            n81 = call <vilib>:"Add State(s) to Queue__JKI_lib_State_Machine.vi"("State(s) in Front (\"\")"="Data: Initialize\nInitialize Core Data\nData: Update Indicators", "State(s) in (\"\")"=w316) -> ("States Out"=w315:string)  [unwired: 13 in]
          }
          frame "Macro: Exit" {
            # "#CSM \"Macro: Exit\"\nExit Macro (This is called once, when the VI exits)"
            n82 = call <vilib>:"Add State(s) to Queue__JKI_lib_State_Machine.vi"("State(s) in Front (\"\")"="//Exit Sub-Modules ", "State(s) at Back (\"\")"="Data: Cleanup\nExit") -> ("States Out"=w318:string)  [unwired: 13 in]
            n83 = call <vilib>:"Add State(s) to Queue__JKI_lib_State_Machine.vi"("State(s) in Front (\"\")"=w318, "State(s) in (\"\")"=w323) -> ("States Out"=w322:string)  [unwired: 13 in]
          }
          frame "---------- API ----------" {
            # "#CSM \"Category Seperator\"\nDo not put any code in this frame."
          }
          frame "API: API1" {
            # "#CSM API Example\nCopy/Rename this case for your own API"
            # "#CSM Response\nConnect this to return the response of your API"
            # "#CSM >> Msg/Rep's CSM >>\nIf you need to tell who triggered this state , use this string. If it's this case itself, this string is \"\"."
            # "#CSM >> Arguments >>\nDeal with the parameter if any"
          }
          frame "API: API2" {
            # "#CSM API Example\nCopy/Rename this case for your own API"
            # "unpack Hex String  to Variant\nif complex parameter is needed."
            n84 = call "CSM - Convert HexStr to Data.vi"("HEX String"=w332) -> ()  [unwired: 7 in, 2 out]
            n85 = disable-structure shown="Disabled" {
              disable-tunnel: [w336 "API2 Response"] -> w331
              frame Disabled {
                # "pack variant to hexstr \nif complex response is needed."
                # "complex Response"
                n86 = call "CSM - Convert Data to HexStr.vi"() -> ("HEX String (0-9,A-F)"=w336:string)  [unwired: 9 in]
              }
              frame Enabled {
              }
            }
          }
          frame "---------- Action ----------" {
            # "#CSM \"Category Seperator\"\nDo not put any code in this frame."
            n87 = call <vilib>:"Add State(s) to Queue__JKI_lib_State_Machine.vi"("State(s) in (\"\")"=w341) -> ("States Out"=w340:string)  [unwired: 14 in]
          }
          frame "Action: action1" {
            # "#CSM \"Internal State\"\nThis category is used for holding internal states"
            n88 = call <vilib>:"Add State(s) to Queue__JKI_lib_State_Machine.vi"("State(s) in (\"\")"=w345) -> ("States Out"=w344:string)  [unwired: 14 in]
          }
          frame "Action: action2" {
            # "#CSM \"Internal State\"\nThis category is used for holding internal states"
            n89 = call <vilib>:"Add State(s) to Queue__JKI_lib_State_Machine.vi"("State(s) in (\"\")"=w349) -> ("States Out"=w348:string)  [unwired: 14 in]
          }
        }
      }
      n90 = flat-sequence {
        tunnel: ["CSM" ("search string")] -> w61
        tunnel: w8 -> [_]
        frame #0 {
        }
      }
      n91 = call-poly "CSM - Filter JKISM String Queue.vi"("States In"=w38) -> ("States Out"=w70:string)  [unwired: 14 in]
      n92 = call-poly "CSM - Filter JKISM String Queue.vi"("States In"=w38) -> ("States Out"=w72:string)  [unwired: 14 in]
      n93 = call-poly "CSM - Filter JKISM String Queue.vi"("States In"=w38) -> ("States Out"=w64:string)  [unwired: 14 in]
      n94 = call-poly "CSM - Filter JKISM String Queue.vi"("States In"=w38) -> ("States Out"=w68:string)  [unwired: 14 in]
      n95 = call-poly "CSM - Filter JKISM String Queue.vi"("States In"=w38) -> ("States Out"=w66:string)  [unwired: 14 in]
      n96 = Search and Replace String(replace all?=TRUE ("replace all? (F)"), input string="Message -> CSM\r\nMessage ->| CSM\r\nAction: Action 1 -> CSM\r\nAction: Action 3 ->| CSM\r\nAPI: API1>>Argument -> CSM\r\nAPI: API1>>Argument ->| CSM", search string=w61, replace string=w7) -> (result string=w57:string)  [unwired: 4 in, 3 out]
      n97 = Concatenate Strings(w38, "\r\n", w57) -> (w59:string)
      n98 = call-poly "CSM - Filter JKISM String Queue.vi"("States In"=w59) -> ("States Out"=w56:string)  [unwired: 14 in]
      n99 = Concatenate Strings("Local States to be filtered:\r\n//Comment A\r\n//Comment A\r\n/*Comment B\r\n//\"->\", \"->|\", \"-@\"\r\nAction: Local State to be filtered\r\n\r\n***SeparationLine***\r\n***SeparationLine***\r\nBroadcast Message>>Argument -> <broadcast>\r\nBroadcast Message>>Argument -> <all>\r\nBroadcast Message>>Argument -> <all>\r\nBroadcast Message>>Argument -> <status>\r\nBroadcast Message>>Argument -> <interrupt>\r\nBroadcast Message>>Argument -> <interupt>\r\nBroadcast Message>>Argument -> <interput>\r\nBroadcast Message>>Argument -> <interput>" ("States Out"), "\r\n", w57) -> (w55:string)
      n100 = flat-sequence {
        tunnel: w7 -> [w74]
        tunnel: w6 -> [_]
        frame #0 {
          n101 = call "CSM - Send Message and Wait for Reply.vi"("Target Module"=w74, "State"="Macro: Exit") -> ()  [unwired: 7 in, 3 out]
        }
      }
      n102 = Equal?(x=w68, y="Local States to be filtered:\r\n//Comment A\r\n//Comment A\r\n/*Comment B\r\n//\"->\", \"->|\", \"-@\"\r\nAction: Local State to be filtered\r\n\r\n***SeparationLine***\r\n***SeparationLine***\r\nMessage -@ CSM\r\nMessage ->| CSM\r\nAction: Action 2 -@ CSM\r\nAction: Action 2 -@ CSM\r\nAction: Action 3 ->| CSM\r\nAPI: API1>>Argument -@ CSM\r\nAPI: API1>>Argument ->| CSM\r\nBroadcast Message>>Argument -> <broadcast>\r\nBroadcast Message>>Argument -> <all>\r\nBroadcast Message>>Argument -> <all>\r\nBroadcast Message>>Argument -> <status>\r\nBroadcast Message>>Argument -> <interrupt>\r\nBroadcast Message>>Argument -> <interupt>\r\nBroadcast Message>>Argument -> <interput>\r\nBroadcast Message>>Argument -> <interput>" ("States In")) -> (x = y?=w27:bool)
      "Filter Async Messages" <- w27
      n103 = Equal?(x=w70, y="Local States to be filtered:\r\n//Comment A\r\n//Comment A\r\n/*Comment B\r\n//\"->\", \"->|\", \"-@\"\r\nAction: Local State to be filtered\r\n\r\n***SeparationLine***\r\n***SeparationLine***\r\nBroadcast Message>>Argument -> <broadcast>\r\nBroadcast Message>>Argument -> <all>\r\nBroadcast Message>>Argument -> <all>\r\nBroadcast Message>>Argument -> <status>\r\nBroadcast Message>>Argument -> <interrupt>\r\nBroadcast Message>>Argument -> <interupt>\r\nBroadcast Message>>Argument -> <interput>\r\nBroadcast Message>>Argument -> <interput>" ("States In")) -> (x = y?=w28:bool)
      "Filter All Messages" <- w28
      n104 = Equal?(x=w66, y="Local States to be filtered:\r\n//Comment A\r\n//Comment A\r\n/*Comment B\r\n//\"->\", \"->|\", \"-@\"\r\nAction: Local State to be filtered\r\n\r\n***SeparationLine***\r\n***SeparationLine***\r\nMessage -> CSM\r\nMessage -@ CSM\r\nAction: Action 1 -> CSM\r\nAction: Action 2 -@ CSM\r\nAction: Action 2 -@ CSM\r\nAPI: API1>>Argument -> CSM\r\nAPI: API1>>Argument -@ CSM\r\nBroadcast Message>>Argument -> <broadcast>\r\nBroadcast Message>>Argument -> <all>\r\nBroadcast Message>>Argument -> <all>\r\nBroadcast Message>>Argument -> <status>\r\nBroadcast Message>>Argument -> <interrupt>\r\nBroadcast Message>>Argument -> <interupt>\r\nBroadcast Message>>Argument -> <interput>\r\nBroadcast Message>>Argument -> <interput>" ("States Out")) -> (x = y?=w26:bool)
      "Filter Async Messages Without Reply" <- w26
      n105 = Equal?(x=w72, y="Message -> CSM\r\nMessage -@ CSM\r\nMessage ->| CSM\r\nAction: Action 1 -> CSM\r\nAction: Action 2 -@ CSM\r\nAction: Action 2 -@ CSM\r\nAction: Action 3 ->| CSM\r\nAPI: API1>>Argument -> CSM\r\nAPI: API1>>Argument -@ CSM\r\nAPI: API1>>Argument ->| CSM\r\nBroadcast Message>>Argument -> <broadcast>\r\nBroadcast Message>>Argument -> <all>\r\nBroadcast Message>>Argument -> <all>\r\nBroadcast Message>>Argument -> <status>\r\nBroadcast Message>>Argument -> <interrupt>\r\nBroadcast Message>>Argument -> <interupt>\r\nBroadcast Message>>Argument -> <interput>\r\nBroadcast Message>>Argument -> <interput>" ("States Out")) -> (x = y?=w29:bool)
      "Fiter Local States" <- w29
      n106 = Equal?(x=w64, y="Local States to be filtered:\r\n//Comment A\r\n//Comment A\r\n/*Comment B\r\n//\"->\", \"->|\", \"-@\"\r\nAction: Local State to be filtered\r\n\r\n***SeparationLine***\r\n***SeparationLine***\r\nMessage -> CSM\r\nMessage ->| CSM\r\nAction: Action 1 -> CSM\r\nAction: Action 3 ->| CSM\r\nAPI: API1>>Argument -> CSM\r\nAPI: API1>>Argument ->| CSM\r\nBroadcast Message>>Argument -> <broadcast>\r\nBroadcast Message>>Argument -> <all>\r\nBroadcast Message>>Argument -> <all>\r\nBroadcast Message>>Argument -> <status>\r\nBroadcast Message>>Argument -> <interrupt>\r\nBroadcast Message>>Argument -> <interupt>\r\nBroadcast Message>>Argument -> <interput>\r\nBroadcast Message>>Argument -> <interput>" ("States Out")) -> (x = y?=w25:bool)
      "Filter Sync Messages" <- w25
      n107 = Equal?(x=w56, y=w55) -> (x = y?=w6:bool)
      "Filter Messages To Non Existing CSMs" <- w6
      n108 = Compound Arithmetic op=AND(w29, w28, w27, w26, w25, w6) -> (w18:bool)
      n109 = Concatenate Strings(w38, "\r\n", "//Comment X\n//Comment X\n/*Comment X\n/*Comment X" ("States Out")) -> (w35:string)
      n110 = call-poly "CSM - Filter JKISM String Queue.vi"("Keep First Matched? (T)"=TRUE, "States In"=w38, "Option"=enum16{"State", "No Comments", "Line"}."State") -> ("States Out"=w46:string)  [unwired: 12 in]
      n111 = call-poly "CSM - Filter JKISM String Queue.vi"("States In"=w38) -> ("States Out"=w52:string)  [unwired: 14 in]
      n112 = call-poly "CSM - Filter JKISM String Queue.vi"("States In"=w38) -> ("States Out"=w54:string)  [unwired: 14 in]
      n113 = call-poly "CSM - Filter JKISM String Queue.vi"("States In"=w38) -> ("States Out"=w50:string)  [unwired: 14 in]
      n114 = call-poly "CSM - Filter JKISM String Queue.vi"("Keep First Matched? (T)"=TRUE, "States In"=w35, "Option"=enum16{"State", "No Comments", "Line"}."No Comments") -> ("States Out"=w37:string)  [unwired: 12 in]
      n115 = call-poly "CSM - Filter JKISM String Queue.vi"("Keep First Matched? (T)"=TRUE, "States In"=w38, "Option"=enum16{"State", "No Comments", "Line"}."Line") -> ("States Out"=w42:string)  [unwired: 12 in]
      n116 = Equal?(x=w54, y="Local States to be filtered:\r\n//Comment A\r\n//Comment A\r\n/*Comment B\r\n//\"->\", \"->|\", \"-@\"\r\nAction: Local State to be filtered\r\n\r\n***SeparationLine***\r\n***SeparationLine***\r\nMessage -> CSM\r\nMessage -@ CSM\r\nMessage ->| CSM\r\nAction: Action 1 -> CSM\r\nAction: Action 2 -@ CSM\r\nAction: Action 2 -@ CSM\r\nAction: Action 3 ->| CSM\r\nAPI: API1>>Argument -> CSM\r\nAPI: API1>>Argument -@ CSM\r\nAPI: API1>>Argument ->| CSM" ("States Out")) -> (x = y?=w24:bool)
      "Fiter Broadcasts" <- w24
      n117 = Equal?(x=w52, y="Local States to be filtered:\r\n//Comment A\r\n//Comment A\r\n/*Comment B\r\n//\"->\", \"->|\", \"-@\"\r\nAction: Local State to be filtered\r\n\r\n***SeparationLine***\r\n***SeparationLine***\r\nMessage -> CSM\r\nMessage -@ CSM\r\nMessage ->| CSM\r\nAction: Action 1 -> CSM\r\nAction: Action 2 -@ CSM\r\nAction: Action 2 -@ CSM\r\nAction: Action 3 ->| CSM\r\nAPI: API1>>Argument -> CSM\r\nAPI: API1>>Argument -@ CSM\r\nAPI: API1>>Argument ->| CSM\r\nBroadcast Message>>Argument -> <interrupt>\r\nBroadcast Message>>Argument -> <interupt>\r\nBroadcast Message>>Argument -> <interput>\r\nBroadcast Message>>Argument -> <interput>" ("States Out")) -> (x = y?=w23:bool)
      "Fiter Status Broadcast" <- w23
      n118 = Equal?(x=w50, y="Local States to be filtered:\r\n//Comment A\r\n//Comment A\r\n/*Comment B\r\n//\"->\", \"->|\", \"-@\"\r\nAction: Local State to be filtered\r\n\r\n***SeparationLine***\r\n***SeparationLine***\r\nMessage -> CSM\r\nMessage -@ CSM\r\nMessage ->| CSM\r\nAction: Action 1 -> CSM\r\nAction: Action 2 -@ CSM\r\nAction: Action 2 -@ CSM\r\nAction: Action 3 ->| CSM\r\nAPI: API1>>Argument -> CSM\r\nAPI: API1>>Argument -@ CSM\r\nAPI: API1>>Argument ->| CSM\r\nBroadcast Message>>Argument -> <broadcast>\r\nBroadcast Message>>Argument -> <all>\r\nBroadcast Message>>Argument -> <all>\r\nBroadcast Message>>Argument -> <status>" ("States Out")) -> (x = y?=w22:bool)
      "Fiter Interrupt Broadcast" <- w22
      n119 = Equal?(x=w46, y="Local States to be filtered:\r\nAction: Local State to be filtered\r\n***SeparationLine***\r\nMessage -> CSM\r\nAction: Action 1 -> CSM\r\nAction: Action 2 -@ CSM\r\nAction: Action 3 ->| CSM\r\nAPI: API1>>Argument -> CSM\r\nBroadcast Message>>Argument -> <broadcast>" ("States Out")) -> (x = y?=w21:bool)
      "Filter Duplicate States(Regardless of async/sync/status/interrupt)" <- w21
      n120 = Equal?(x=w42, y="Local States to be filtered:\r\n//Comment A\r\n/*Comment B\r\n//\"->\", \"->|\", \"-@\"\r\nAction: Local State to be filtered\r\n***SeparationLine***\r\nMessage -> CSM\r\nMessage -@ CSM\r\nMessage ->| CSM\r\nAction: Action 1 -> CSM\r\nAction: Action 2 -@ CSM\r\nAction: Action 3 ->| CSM\r\nAPI: API1>>Argument -> CSM\r\nAPI: API1>>Argument -@ CSM\r\nAPI: API1>>Argument ->| CSM\r\nBroadcast Message>>Argument -> <broadcast>\r\nBroadcast Message>>Argument -> <all>\r\nBroadcast Message>>Argument -> <status>\r\nBroadcast Message>>Argument -> <interrupt>\r\nBroadcast Message>>Argument -> <interupt>\r\nBroadcast Message>>Argument -> <interput>" ("States Out")) -> (x = y?=w20:bool)
      "Filter Duplicate Lines" <- w20
      n121 = Equal?(x=w37, y="Local States to be filtered:\r\nAction: Local State to be filtered\r\n***SeparationLine***\r\nMessage -> CSM\r\nMessage -@ CSM\r\nMessage ->| CSM\r\nAction: Action 1 -> CSM\r\nAction: Action 2 -@ CSM\r\nAction: Action 3 ->| CSM\r\nAPI: API1>>Argument -> CSM\r\nAPI: API1>>Argument -@ CSM\r\nAPI: API1>>Argument ->| CSM\r\nBroadcast Message>>Argument -> <broadcast>\r\nBroadcast Message>>Argument -> <all>\r\nBroadcast Message>>Argument -> <status>\r\nBroadcast Message>>Argument -> <interrupt>\r\nBroadcast Message>>Argument -> <interupt>\r\nBroadcast Message>>Argument -> <interput>" ("States Out")) -> (x = y?=w19:bool)
      "Filter Duplicate Lines No Comments" <- w19
      n122 = Compound Arithmetic op=AND(w24, w23, w22, w21, w20, w19) -> (w17:bool)
      n123 = And(x=w18, y=w17) -> (x .and. y?=w16:bool)
      n124 = call-dynamic "passIf.vi"("error in (no error)"=w31, "message (\"\")"="1. The first line comment can not be filtered out.\n2. Add feature for advanced state filtering.\nSee Github Issue #580" ("message (\"\")"), "pass"=w16, "TestCase in"=w32) -> ("error out"=w30:errorcluster, "TestCase out"=w33:refnum<class "testcase-CSMManagementAPI.lvclass">)  [unwired: 6 in]
    }
    frame Disabled {
      # "skip test result while test is under development"
      n125 = call <vilib>:"skip.vi"("error in (no error)"=w350, "TestCase in"=w353) -> ("error out"=w352:errorcluster, "TestCase out"=w351:refnum<class "testcase-CSMManagementAPI.lvclass">)  [unwired: 8 in]
    }
  }
  "error out" <- w4
  "TestCase out" <- w2
